vi "GT_Open.vi"() -> (0 "rtn_Out":cluster{"rtn":i16, "Func":string})   [LabVIEW 2014]
uses:
  VC6/gts.dll
panel:
  in  "rtn_In":cluster{"rtn":i16, "Func":string}
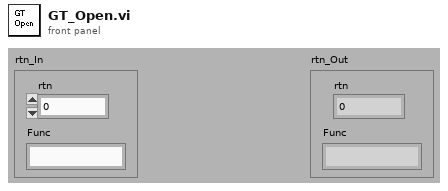
[diagram p1: front panel]
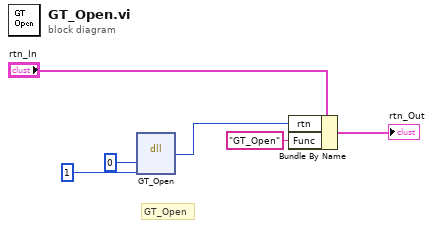
[diagram p0: block diagram]
diagram:
  # "GT_Open"
  n1 = dll-call lib="PTH2Fabs DNewGTS AC-800LWin7版源程序-20170926gts85VC6gts.dll" fn="GT_Open"("Channel"=i16 0, "Param"=i16 1) -> ("rtn"=w3:i16)  [unwired: 5 in, 2 out]
  n2 = Bundle By Name(cluster="rtn_In", "rtn"=w3, "Func"="GT_Open") -> (→"rtn_Out":cluster{"rtn":i16, "Func":string})
